vi "get_polarity_values.vi"(0 "reference (in)":i32, 5 "error in (no error)":errorcluster) -> (14 "reference (dup)":i32, 16 "polarity_items":T1[](array[typedef]), 17 "raw_polarity_value":string, 19 "error out":errorcluster)   [LabVIEW 2012]
doc: "This VI reads the Polarity settings for (7) items in the attached USB device. Those items are:\n\n- DIRECTION\n- LIMIT\n- HOME\n- DIGITAL OUTPUT\n- DIGITAL INPUT\n- ENABLE OUTPUT\n- JUMP TO LINE 0 ON ERROR\n\nAll polarity settings will appear in the output array along with their corresponding states.\nProduced By:\n\nChristopher Lemieux\nKod Integrations, LLC\n4835 Marianne Drive\nMount Airy, MD 21771\nhttp://www.kodintegrations.com\nemail: clemieux@kodintegrations.com\nphone: (240) 687-1288"
uses:
  support/controls/polarity_item_group.ctl
  support/controls/polarity_items.ctl
  main_functions/commands.ctl
  support/controls/simple_actions.ctl
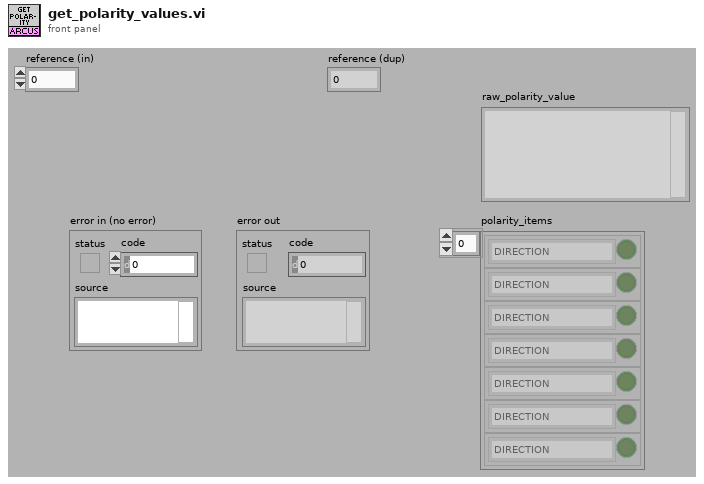
[diagram p1: front panel]
types:
  T1 = typedef "polarity_item_group.ctl" = cluster{"item":T2, "status":bool}
  T2 = typedef "polarity_items.ctl" = enum16{"DIRECTION", "LIMIT", "HOME", "DIG_OUT", "DIG_IN", "ENABLE_OUT", "JUMP_ERR"}
  T3 = typedef "simple_actions.ctl" = enum16{"from", "to"}
  T4 = typedef "commands.ctl" = enum16{"clear error", "constant jog(-)", "constant jog(+)", "get acceleration", "get actual current", "get device id", "get digital input status", "get digial inputs status", "get dig output status", "get digital outputs status", "get firmware ver", "get high speed", "get idle current", "get low speed", "get micro step", "get motor status", "get move mode", "get polarity", "get position", "get product id", "get power status", "get run current", "get status", "home(-)", "home(+)", "move to position", "power down", "power up", "set acceleration", "set device id", "set digital output", "set digital outputs", "set high speed", "set idle current", "set low speed", "set move mode absolute", "set move mode increment", "set polarity", "set position", "set run current", "stop immediate", "stop slow", "store to memory"}
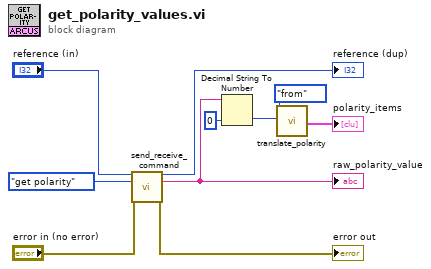
[diagram p0: block diagram]
diagram:
  n1 = call "send_receive_command.vi"("reference (in)"="reference (in)", "command"=commands."get polarity", "error in (no error)"="error in (no error)") -> ("reference (dup)"=→"reference (dup)":i32, "read_string"=w7:string, "error out"=→"error out":errorcluster)  [unwired: 8 in, 2 out]
  "raw_polarity_value" <- w7
  n2 = Decimal String To Number(string=w7, default (0L)=u32 0 ("default (0 I32)")) -> (number=w4:u32)  [unwired: 1 in, 1 out]
  n3 = call "translate_polarity.vi"("simple_actions"=simple_actions."from", "polarity_value (in)"=w4) -> ("polarity_items (out)"=→"polarity_items":T1[])  [unwired: 16 in, 1 out]
